vi "Untitled 2.vi"() -> ()   [LabVIEW 2018]
uses:
  #include/Global textParse.vi
panel:
  in  "y":bool
  in  "Inspection Point":string(combo)
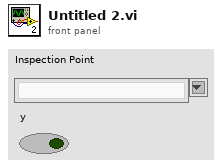
[diagram p1: front panel]
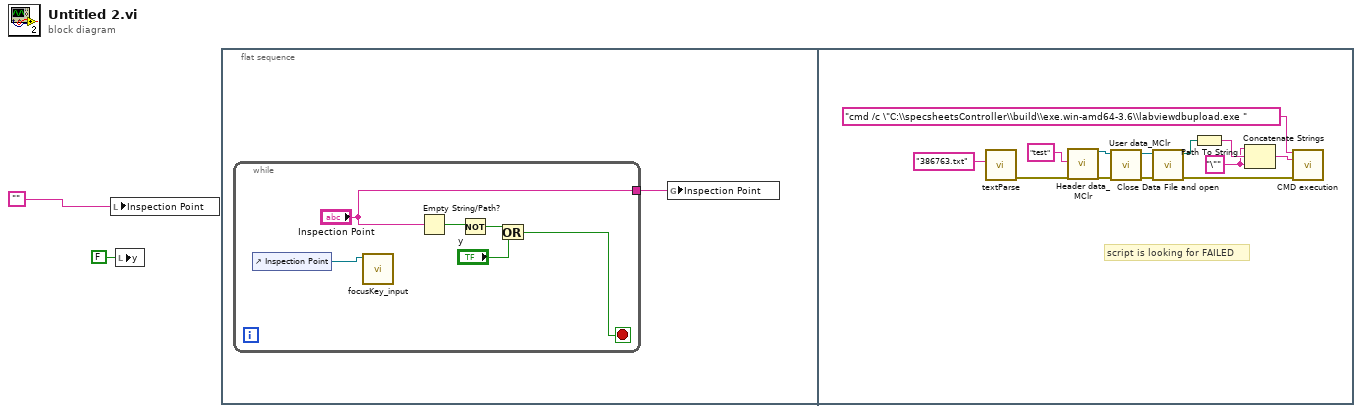
[diagram p0: block diagram]
diagram:
  n1 = local write "Inspection Point"("") -> ()
  n2 = local write "y"(FALSE ("y")) -> ()
  n3 = flat-sequence {
    frame #0 {
      n4 = while {
        tunnel: ["Inspection Point"] -> w3
        stop <- w5 stop-if-true
        n5 = control-ref of="Inspection Point"() -> (w9:refnum<vi>)
        n6 = call "focusKey_input.vi"("reference"=w9) -> ()  [unwired: 10 in, 1 out]
        n7 = Empty String/Path?(string/path="Inspection Point") -> (empty?=w8:bool)
        n8 = Not(x=w8) -> (.not. x?=w7:bool)
        n9 = Or(x=w7, y="y") -> (x .or. y?=w5:bool)
      }
      n10 = global write "Global textParse.vi" "Inspection Point"(w3) -> ()
    }
    frame #1 {
      w13 = "\""
      # "script is looking for FAILED"
      n11 = call "textParse.vi"("file name"="386763.txt") -> ("error out"=w16:errorcluster)  [unwired: 8 in, 2 out]
      n12 = call "Header data_MClr.vi"("file name"="test", "Error In"=w16) -> ("refnum out"=w14:refnum<file>, "error out"=w15:errorcluster)  [unwired: 16 in]
      n13 = call "User data_MClr.vi"("Error In"=w15, "refnum in"=w14) -> ("error out"=w17:errorcluster, "refnum out"=w18:refnum<file>)  [unwired: 6 in]
      n14 = call "Close Data File and open.vi"("error in"=w17, "File Refnum In"=w18) -> ("error out"=w19:errorcluster, "path"=w20:path)  [unwired: 8 in]
      n15 = Path To String(path=w20) -> (string=w21:string)
      n16 = Concatenate Strings(w13, w21, w13) -> (w22:string)
      n17 = call "CMD execution.vi"(".exe"="cmd /c \"C:\\specsheetsController\\build\\exe.win-amd64-3.6\\labviewdbupload.exe ", "file path"=w22, "error in (no error)"=w19) -> ()  [unwired: 11 in, 2 out]
    }
  }
